vi "PRL STR Convert CSG Array to Strings.vi"(10 "Angle View?":bool, 11 "Phasor":csg[](array[numeric])) -> (3 "Strings":string[](array[string]))   [LabVIEW 2013, in "PMU Recorder Light.lvlib"]
uses:
  PMU Recorder Light.lvlib
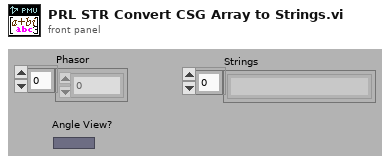
[diagram p1: front panel]
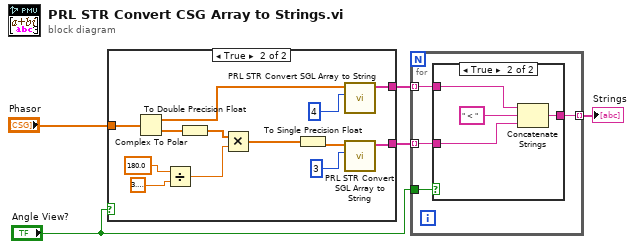
[diagram p0: block diagram]
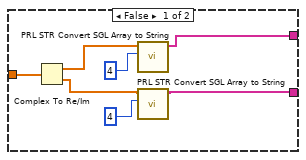
[diagram p2: hidden frame]
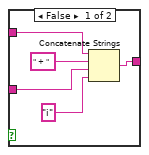
[diagram p3: hidden frame]
diagram:
  n1 = case shown="True" "Angle View?" {
    tunnel: "Phasor" -> [w12 w23]
    tunnel: [w11 w18] -> w4
    tunnel: [w6 w17] -> w3
    frame False {
      n2 = Complex To Re/Im(x + iy=w12) -> (x=w10:sgl[], y=w7:sgl[])
      n3 = call "PRL STR Convert SGL Array to String.vi"("Precision"=4, "Values"=w10) -> ("Strings"=w11:string[])  [unwired: 9 in]
      n4 = call "PRL STR Convert SGL Array to String.vi"("Precision"=4, "Values"=w7) -> ("Strings"=w6:string[])  [unwired: 9 in]
    }
    frame True {
      n5 = Complex To Polar(r * e^(i*theta)=w23) -> (r=w13:sgl[], theta=w22:sgl[])
      n6 = Divide(x=180.0, y=3.141592653589793) -> (x/y=w21:dbl)
      n7 = To Double Precision Float(number=w22) -> (double precision float=w20:dbl[])
      n8 = Multiply(x=w20, y=w21) -> (x*y=w19:dbl[])
      n9 = To Single Precision Float(number=w19) -> (single precision float=w16:sgl[])
      n10 = call "PRL STR Convert SGL Array to String.vi"("Precision"=4, "Values"=w13) -> ("Strings"=w18:string[])  [unwired: 9 in]
      n11 = call "PRL STR Convert SGL Array to String.vi"("Precision"=3, "Values"=w16) -> ("Strings"=w17:string[])  [unwired: 9 in]
    }
  }
  n12 = for {
    tunnel: w4 -> [w29] mode=indexing
    tunnel: w3 -> [w28] mode=indexing
    tunnel: [w27] -> w2 mode=indexing
    tunnel: "Angle View?" -> [w26]
    n13 = case shown="True" w26 {
      tunnel: w29 -> [w33 w37]
      tunnel: w28 -> [w32 w36]
      tunnel: [w30 w35] -> w27
      frame False {
        n14 = Concatenate Strings(w33, " + " ("string"), w32, "i" ("string")) -> (w30:string)
      }
      frame True {
        n15 = Concatenate Strings(w37, " < " ("string"), w36) -> (w35:string)
      }
    }
  }
  "Strings" <- w2
